vi "p2.vi"() -> ()   [LabVIEW 2025, in "d8.lvlib"]
uses:
  d8.lvlib
  2f95b5ca-4bd9-4e55-813b-cc9c1675ecd6.vi
  AOC/AOC.lvlib
panel:
  in  "Example":string="RL\n\nAAA = (BBB, CCC)\nBBB = (DDD, EEE)\nCCC = (ZZZ, GGG)\nDDD = (DDD, DDD)\nEEE = (EEE, EEE)\nGGG = (GGG, GGG)\nZZZ = (ZZZ, ZZZ)"
  in  "Example 2":bool
  out "Answer":i64=12169
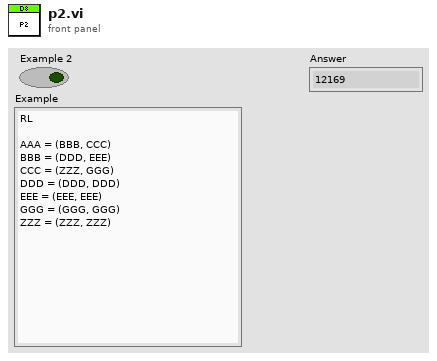
[diagram p1: front panel]
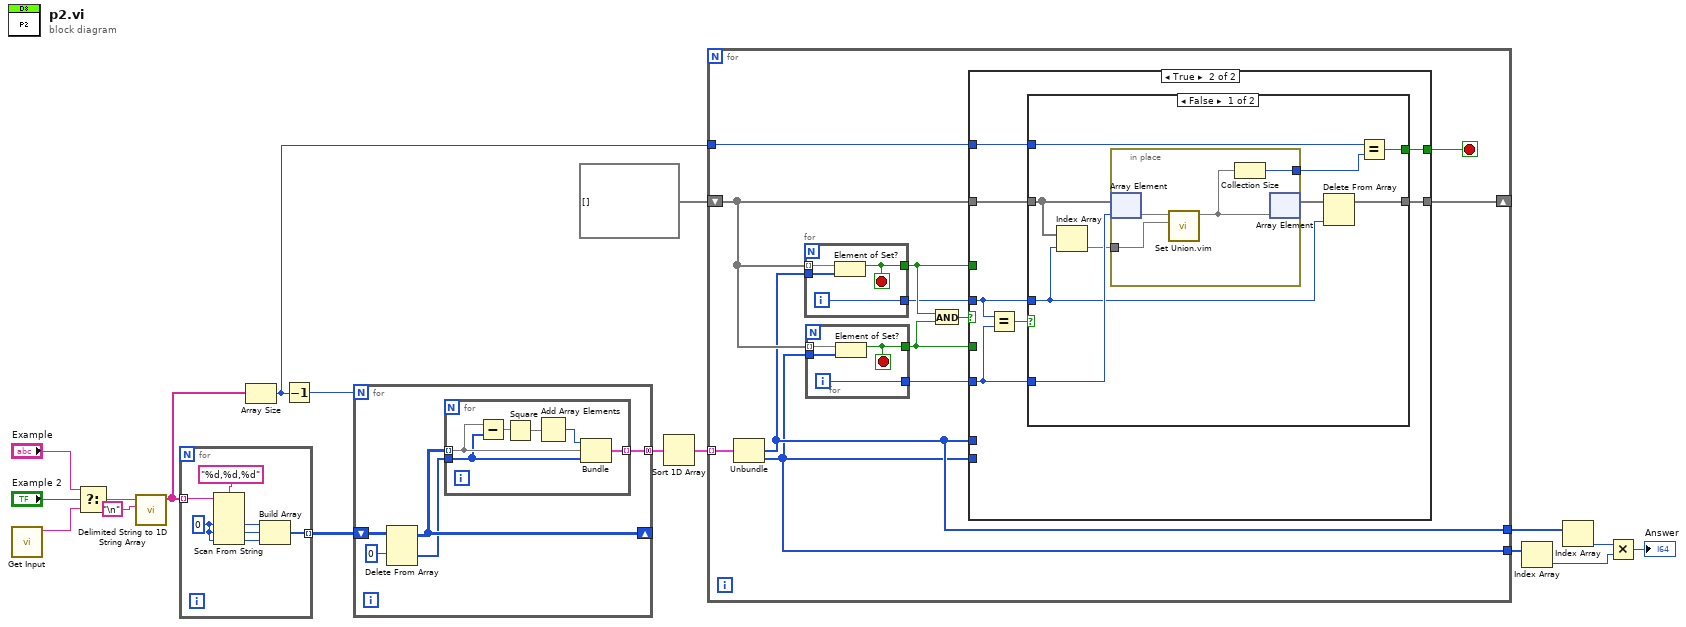
[diagram p0: block diagram]
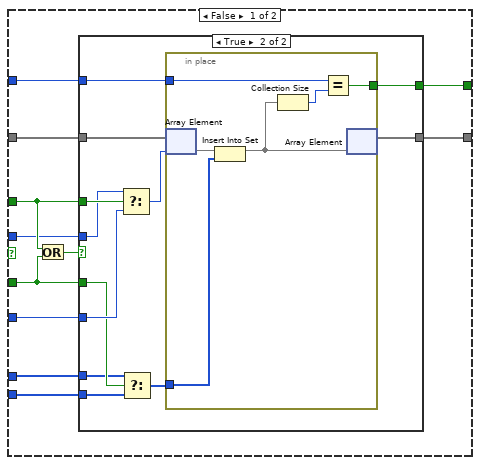
[diagram p2: hidden frame]
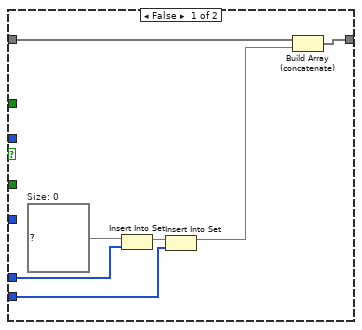
[diagram p3: hidden frame]
diagram:
  n1 = call "Get Input.vi"() -> ("Input"=w17:string)  [unwired: 11 in]
  n2 = Select(t="Example", s="Example 2", f=w17) -> (s? t:f=w16:string)
  n3 = call <vilib>:"Delimited String to 1D String Array.vi"("delimiter"="\n", "delimited string"=w16) -> ("string array"=w13:string[])  [unwired: 9 in]
  n4 = for {
    tunnel: w13 -> [w24] mode=indexing
    tunnel: [w19] -> w12 mode=indexing
    w18 = i64 0 ("default value 14")
    n5 = Scan From String(format string="%d,%d,%d", input string=w24, default 1=w18, default 2=w18, default 3=w18) -> (output 1=w22:i64, output 2=w21:i64, output 3=w20:i64)  [unwired: 2 in, 3 out]
    n6 = Build Array(w22, w21, w20) -> (w19:i64[])
  }
  n7 = Array Size(array=w13) -> (size(s)=w6:i32)
  n8 = Decrement(x=w6) -> (x-1=w9:i32)
  n9 = for {
    N: w9 -> [_]
    shift-right: [w27] -> _
    shift-left: w12 -> [w29]
    tunnel: [w25] -> w11 mode=concatenating
    n10 = Delete From Array(array=w29, index (row)=0) -> (deleted portion=w26:i64[], array with subset deleted=w27:i64[][])  [unwired: 2 in]
    n11 = for {
      tunnel: w27 -> [w35] mode=indexing
      tunnel: w26 -> [w34]
      tunnel: [w30] -> w25 mode=indexing
      n12 = Subtract(x=w35, y=w34) -> (x-y=w33:i64[])
      n13 = Square(x=w33) -> (x^2=w32:i64[])
      n14 = Add Array Elements(numeric array=w32) -> (sum=w31:i64)
      n15 = Bundle("default value 14"=w31, w35, w34) -> (w30:cluster{"default value 14":i64, i64[], i64[]})  [unwired: 1 in]
    }
  }
  n16 = Sort 1D Array(array=w11) -> (sorted array=w7:cluster{"default value 14":i64, i64[], i64[]}[])
  n17 = for {
    shift-right: [w40] -> _
    shift-left: set{i64[]}[] [] -> [w41]
    tunnel: w7 -> [w47] mode=indexing
    tunnel: w6 -> [w39]
    tunnel: [w37] -> w5
    tunnel: [w36] -> w4
    stop <- w38 stop-if-true
    n18 = Unbundle(w47) -> (w37:i64[], w36:i64[])  [unwired: 1 out]
    n19 = for {
      tunnel: w37 -> [w111]
      tunnel: w41 -> [w112] mode=indexing
      tunnel: [w110] -> w45
      tunnel: [w109] -> w43
      i -> [w109]
      stop <- w110 stop-if-true
      n20 = Element of Set?(10:w111, 11:w112) -> (3:w110:bool)
    }
    n21 = for {
      tunnel: w36 -> [w107]
      tunnel: w41 -> [w108] mode=indexing
      tunnel: [w106] -> w44
      tunnel: [w105] -> w42
      i -> [w105]
      stop <- w106 stop-if-true
      n22 = Element of Set?(10:w107, 11:w108) -> (3:w106:bool)
    }
    n23 = And(x=w45, y=w44) -> (x .and. y?=w46:bool)
    n24 = case shown="True" w46 {
      tunnel: w45 -> [w57 _]
      tunnel: w44 -> [w53 _]
      tunnel: w43 -> [w55 w89]
      tunnel: w42 -> [w56 w88]
      tunnel: w41 -> [w54 w87]
      tunnel: [w50 w86] -> w40
      tunnel: w36 -> [w51 _]
      tunnel: w37 -> [w52 _]
      tunnel: w39 -> [w49 w85]
      tunnel: [w48 w84] -> w38
      frame False {
        n25 = Or(x=w57, y=w53) -> (x .or. y?=w58:bool)
        n26 = case shown="True" w58 {
          tunnel: w57 -> [_ w77]
          tunnel: w56 -> [_ w76]
          tunnel: w55 -> [_ w75]
          tunnel: w54 -> [w65 w74]
          tunnel: w53 -> [_ w72]
          tunnel: w52 -> [w60 w71]
          tunnel: w51 -> [w59 w70]
          tunnel: [w64 w68] -> w50
          tunnel: w49 -> [_ w67]
          tunnel: [_ w66] -> w48
          frame False {
            w61 = set{i64[]} {}  # Size: 0
            n27 = Insert Into Set(10:w60, 11:w61) -> (3:w62:set{i64[]})  [unwired: 1 out]
            n28 = Insert Into Set(10:w59, 11:w62) -> (3:w63:set{i64[]})  [unwired: 1 out]
            n29 = Build Array (concatenate)(w65, w63) -> (w64:set{i64[]}[])
          }
          frame True {
            n30 = Select(t=w75, s=w77, f=w76) -> (s? t:f=w73:i32)
            n31 = Select(t=w71, s=w72, f=w70) -> (s? t:f=w69:i64[])
            n32 = in-place {
              in-place-border: w69 -> [w82]
              in-place-border: w67 -> [w79]
              in-place-border: [w78] -> w66
              n33 = in-place-array #1(w74, w73) -> (w83:set{i64[]})
              n34 = Insert Into Set(10:w82, 11:w83) -> (3:w81:set{i64[]})  [unwired: 1 out]
              n35 = Collection Size(1:w81) -> (0:w80:i32)
              n36 = Equal?(x=w79, y=w80) -> (x = y?=w78:bool)
              n37 = in-place-array #1(w81) -> (w68:set{i64[]}[])  [unwired: 1 out]
            }
          }
        }
      }
      frame True {
        n38 = Equal?(x=w89, y=w88) -> (x = y?=w90:bool)
        n39 = case shown="False" w90 {
          tunnel: w89 -> [w95 _]
          tunnel: w88 -> [w99 _]
          tunnel: w87 -> [w97 w104]
          tunnel: [w94 w104] -> w86
          tunnel: w85 -> [w93 _]
          tunnel: [w91 _] -> w84
          frame False {
            n40 = Index Array(array=w97, index=w95) -> (element=w96:set{i64[]})
            n41 = in-place {
              in-place-border: w96 -> [w102]
              in-place-border: [w100] -> w92
              n42 = in-place-array #2(w97, w99) -> (w103:set{i64[]})
              n43 = call "Set Union.vim"("set 2"=w102, "set 1"=w103) -> ("union"=w101:set{i64[]})  [unwired: 9 in]
              n44 = Collection Size(1:w101) -> (0:w100:i32)
              n45 = in-place-array #2(w101) -> (w98:set{i64[]}[])  [unwired: 1 out]
            }
            n46 = Delete From Array(array=w98, index=w95) -> (array with subset deleted=w94:set{i64[]}[])  [unwired: 1 in, 1 out]
            n47 = Equal?(x=w93, y=w92) -> (x = y?=w91:bool)
          }
          frame True {
          }
        }
      }
    }
  }
  n48 = Index Array(array=w4) -> (element=w2:i64)  [unwired: 1 in]
  n49 = Index Array(array=w5) -> (element=w3:i64)  [unwired: 1 in]
  n50 = Multiply(x=w3, y=w2) -> (x*y=→"Answer":i64)
